vi "Create_Trajectory_Units_To_Meters.vi"(6 "Units Selector":T1, 11 "Units":dbl) -> (3 "Meters":dbl)   [LabVIEW 2019]
doc: "Convert given units to Meter"
uses:
  <vilib>/Rock Robotics/WPI/ThirdParty/JAS_Junk/TrajLib/Trajectory_Library.lvlib
  TrajCreateUnitsENUM.ctl
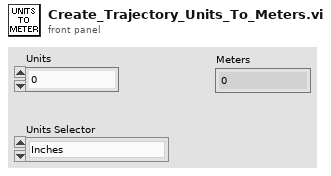
[diagram p1: front panel]
types:
  T1 = typedef "TrajCreateUnitsENUM.ctl" = enum16{"Inches", "Feet", "Centimeters", "Meters"}
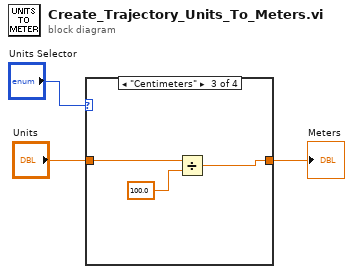
[diagram p0: block diagram]
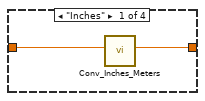
[diagram p2: hidden frame]
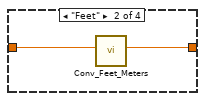
[diagram p3: hidden frame]
diagram:
  n1 = case shown="\"Centimeters\"" "Units Selector" {
    tunnel: [w4 w6 w8 w11] -> w3
    tunnel: "Units" -> [w5 w7 w10 w11]
    frame "Inches" {
      n2 = call <vilib>:"Conv_Inches_Meters.vi"("INCH"=w5) -> ("Meters"=w4:dbl)  [unwired: 10 in]
    }
    frame "Feet" {
      n3 = call <vilib>:"Conv_Feet_Meters.vi"("Feet"=w7) -> ("Meters"=w6:dbl)  [unwired: 10 in]
    }
    frame "Centimeters" {
      n4 = Divide(x=w10, y=100.0) -> (x/y=w8:dbl)
    }
    frame "Meters" {
    }
  }
  "Meters" <- w3
